vi "Test_Surge_Commandlist.vi"() -> ()   [LabVIEW 2013, in "VI-Test.lvlib"]
uses:
  lib/VI-Test.lvlib
  classes/Tests/Surge/Surge.lvclass
panel:
  out "wait":i32[](array[numeric])=[0, 30000, 0, 0]
  out "timeout":u32[](array[numeric])
  out "parameters":string[][](table)
  out "Commandlist":string
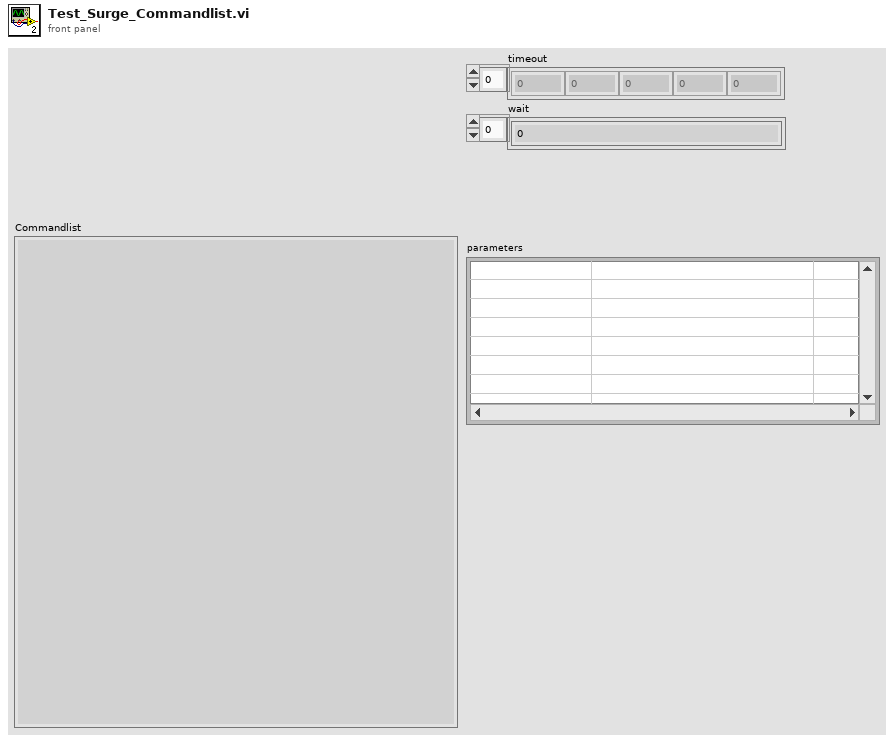
[diagram p1: front panel]
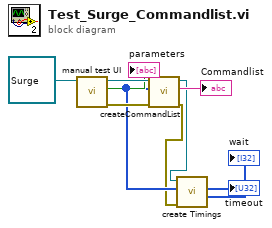
[diagram p0: block diagram]
diagram:
  n1 = call-dynamic "manual test UI.vi"("Surge Eingang"=refnum<class "Surge.lvclass"> refnum) -> ("error out"=w10:errorcluster, "abbrechen"=→"parameters":bool, "Parameters"=w5:u32[], "Surge Ausgang"=w9:refnum<class "Surge.lvclass">)  [unwired: 7 in]
  n2 = call-dynamic "createCommandList.vi"("error in (no error)"=w10, "Parameters"=w5, "Surge in"=w9) -> ("error out"=w3:errorcluster, "Commandlist"=→"Commandlist":string, "Surge out"=w4:refnum<class "Surge.lvclass">)  [unwired: 6 in]
  n3 = call-dynamic "create Timings.vi"("error in (no error)"=w3, "Parameters"=w5, "Surge in"=w4) -> ("wait"=→"wait":i32[], "timeout"=→"timeout":u32[])  [unwired: 5 in, 2 out]
